vi "I2C Example.vi"() -> ()   [LabVIEW 2021]
uses:
  src/Typedef/Link Types.ctl
  src/pcap Parse and Build.lvclass
  <vilib>/CIF Foundation/CIF Utilities/Time/Time_CIF_U.lvlib
panel:
  out "LabVIEW Time (s)":timestamp
  out "Read":bool
  out "Bus":u8 format="%.0x"
  out "7 bit Address":u8 format="%.0x"
  out "Payload":u8[](array[numeric]) format="%.0x"
  out "File":string
  in  "file path (use dialog)":path
  out "error out":errorcluster
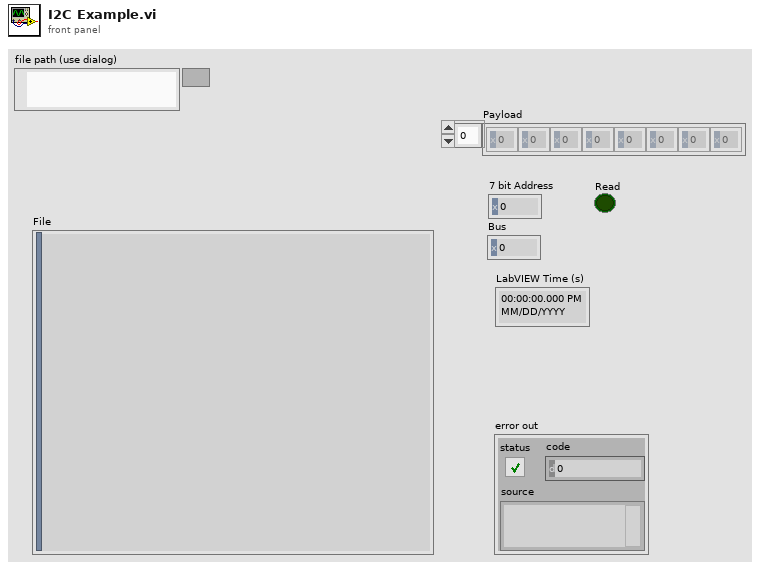
[diagram p1: front panel]
types:
  T1 = typedef "pcap Parse and Build.lvclass/Link Types.ctl" = enum16{"Override", "Ethernet", "Socket CAN", "I2C Linux"}
  T2 = enum16{"open", "replace", "create", "open or create", "replace or create", "replace or create with confirmation"}
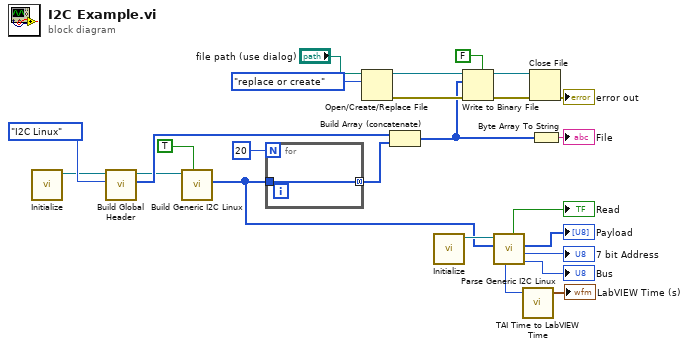
[diagram p0: block diagram]
diagram:
  n1 = call "Initialize.vi"() -> ("pcap Parse and Build out"=w12:refnum<class "pcap Parse and Build.lvclass">)  [unwired: 11 in]
  n2 = call "Build Global Header.vi"("Link Types"=Link_Types."I2C Linux", "pcap Parse and Build in"=w12) -> ("Global Header"=w14:u8[], "pcap Parse and Build out"=w10:refnum<class "pcap Parse and Build.lvclass">)  [unwired: 7 in, 1 out]
  n3 = call "Build Generic I2C Linux.vi"("Read"=TRUE, "pcap Parse and Build in"=w10) -> ("I2C Packet"=w5:u8[])  [unwired: 8 in, 1 out]
  n4 = for {
    N: 20 -> [_]
    tunnel: w5 -> [w26]
    tunnel: [w26] -> w11 mode=concatenating
  }
  n5 = Open/Create/Replace File(file path (use dialog)="file path (use dialog)", operation (0:open)=T2."replace or create") -> (refnum out=w23:refnum<file>, error out=w24:errorcluster)  [unwired: 4 in, 1 out]
  n6 = Build Array (concatenate)(w14, w11) -> (w15:u8[])
  n7 = call "Initialize.vi"() -> ("pcap Parse and Build out"=w6:refnum<class "pcap Parse and Build.lvclass">)  [unwired: 11 in]
  n8 = Write to Binary File(file (use dialog)=w23, data=w15, error in=w24, 5:FALSE ("prepend array or string size? (T)")) -> (refnum out=w20:refnum<file>, error out=w19:errorcluster)  [unwired: 2 in, 1 out]
  n9 = call "Parse Generic I2C Linux.vi"("Bytes in"=w5, "pcap Parse and Build in"=w6) -> ("Bus"=→"Bus":u8, "7 bit Address"=→"7 bit Address":u8, "Payload"=→"Payload":u8[], "Read"=→"Read":bool, "TAI Time (ns)"=w3:i64)  [unwired: 4 in, 1 out]
  n10 = call <vilib>:"TAI Time to LabVIEW Time.vi"("TAI Time (ns)"=w3) -> ("LabVIEW Time (s)"=→"LabVIEW Time (s)":timestamp)  [unwired: 4 in]
  n11 = Close File(refnum=w20, error in=w19) -> (error out=→"error out":errorcluster)  [unwired: 1 out]
  n12 = Byte Array To String(unsigned byte array=w15) -> (string=→"File":string)
